vi "Check for Invalid FIFO Configuration.vi"(10 "Desired FIFO":bool, 11 "Region":T1) -> (3 "Invalid FIFO Configuration":bool)   [LabVIEW 2015, in "NI_AWS_SQS.lvclass"]
uses:
  NI_AWS_SQS.lvclass
  Core/Region.ctl
  Core/NI_AWS_Core.lvclass
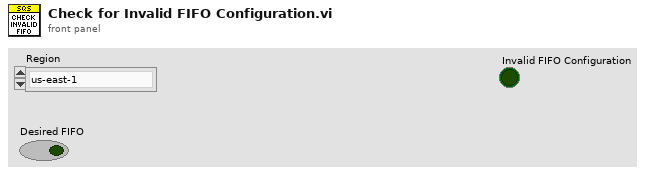
[diagram p1: front panel]
types:
  T1 = typedef "NI_AWS_Core.lvclass/Region.ctl" = enum16{"us-east-1", "us-east-2", "us-west-1", "us-west-2", "ap-northeast-1", "ap-northeast-2", "ap-southeast-1", "ap-southeast-2", "ca-central-1", "eu-central-1", "eu-west-1", "eu-west-2", "sa-east-1"}
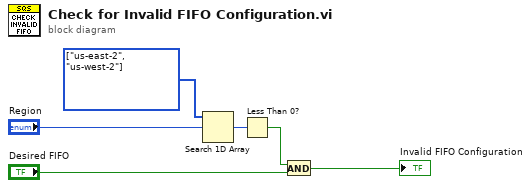
[diagram p0: block diagram]
diagram:
  w3 = T1[] [enum."us-east-2", enum."us-west-2"] items=["us-east-1", "us-east-2", "us-west-1", "us-west-2", "ap-northeast-1", "ap-northeast-2", "ap-southeast-1", "ap-southeast-2", "ca-central-1", "eu-central-1", "eu-west-1", "eu-west-2", "sa-east-1"] ("1D array")
  n1 = Search 1D Array(1D array=w3, element="Region") -> (index of element=w4:i32)  [unwired: 1 in]
  n2 = Less Than 0?(x=w4) -> (x < 0?=w5:bool)
  n3 = And(x=w5, y="Desired FIFO") -> (x .and. y?=→"Invalid FIFO Configuration":bool)
